vi "PLC Rotate Unpuck.vi"(7 "PVT in":T1={"Mode"=1, "PV Angle"=0.0, "SP_Angle"=0.0, "Rotate Angle"=0.0, "Timeout"=0.0, "Start"=FALSE, "Home"=FALSE} {"Rotate Angle" format="%.1f"; "SP_Angle" format="%.1f"; "PV Angle" format="%.2f"; "Mode" items=["Поворот"=1, "Качение"=2]}, 11 "register values":u16[](array[numeric])) -> (3 "Rotate":T1={"Mode"=1, "PV Angle"=0.0, "SP_Angle"=0.0, "Rotate Angle"=0.0, "Timeout"=0.0, "Start"=FALSE, "Home"=FALSE} {"Rotate Angle" format="%.1f"; "SP_Angle" format="%.1f"; "PV Angle" format="%.2f"; "Mode" items=["Поворот"=1, "Качение"=2]})   [LabVIEW 2018, in "Drive.lvlib"]
uses:
  Drive.lvlib
  Rotation Control Type.ctl
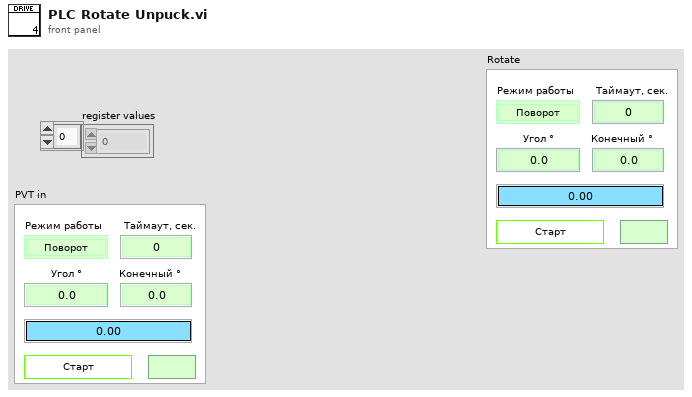
[diagram p1: front panel]
types:
  T1 = typedef "Drive.lvlib/Rotation Control Type.ctl" = cluster{"Mode":u16, "PV Angle":dbl, "SP_Angle":dbl, "Rotate Angle":dbl, "Timeout":dbl, "Start":bool, "Home":bool}
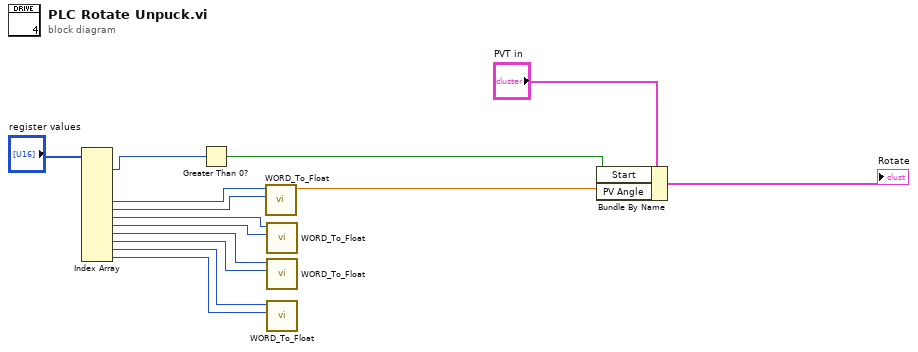
[diagram p0: block diagram]
diagram:
  n1 = Index Array(array="register values") -> (element #1=w1:u16, element #5=w10:u16, element #6=w9:u16, element #7=w8:u16, element #8=w7:u16, element #9=w6:u16, element #10=w5:u16, element #11=w3:u16, element #12=w2:u16)  [unwired: 12 in, 3 out]
  n2 = Greater Than 0?(x=w1) -> (x > 0?=w12:bool)
  n3 = call "WORD_To_Float.vi"("second_Word"=w9, "first_Word"=w10) -> ("output_Float"=w4:sgl)  [unwired: 9 in]
  n4 = call "WORD_To_Float.vi"("second_Word"=w7, "first_Word"=w8) -> ()  [unwired: 9 in, 1 out]
  n5 = call "WORD_To_Float.vi"("second_Word"=w5, "first_Word"=w6) -> ()  [unwired: 9 in, 1 out]
  n6 = call "WORD_To_Float.vi"("second_Word"=w2, "first_Word"=w3) -> ()  [unwired: 9 in, 1 out]
  n7 = Bundle By Name(cluster="PVT in", "Start"=w12, "PV Angle"=w4) -> (→"Rotate":T1)
